vi "Agilent SNA Preset.vi"(7 "Agilent SNA & SWP":T1, 8 "error in (no error)":errorcluster, 11 "VISA Resource Names":T2) -> (0 "error out":errorcluster, 3 "dup VISA Resource Names":T2)   [LabVIEW 2011]
uses:
  TypeDefs/Agilent SNA VISA.ctl
  TypeDefs/Agilent SNA Instrument Info.ctl
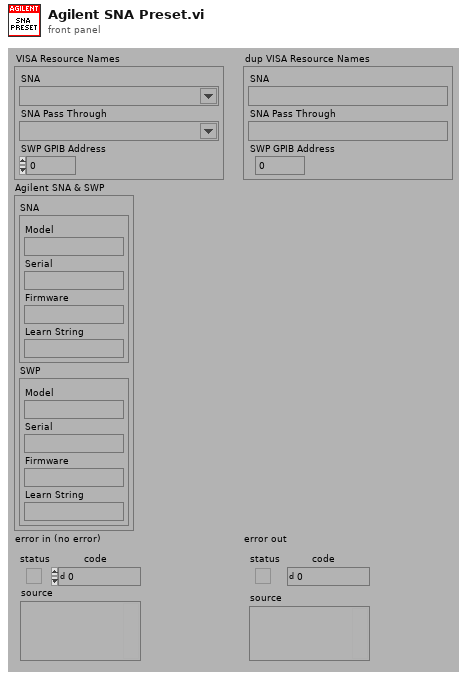
[diagram p1: front panel]
types:
  T1 = typedef "Agilent SNA Instrument Info.ctl" = cluster{"SNA":cluster{"Model":string, "Serial":string, "Firmware":string, "Learn String":string}, "SWP":cluster{"Model":string, "Serial":string, "Firmware":string, "Learn String":string}}
  T2 = typedef "Agilent SNA VISA.ctl" = cluster{"SNA":refnum<visa-resource-name>, "SNA Pass Through":refnum<visa-resource-name>, "SWP GPIB Address":i32}
  T3 = typedef "Agilent SNA Model.ctl" = enum16{"Not Supported", "8757X"}
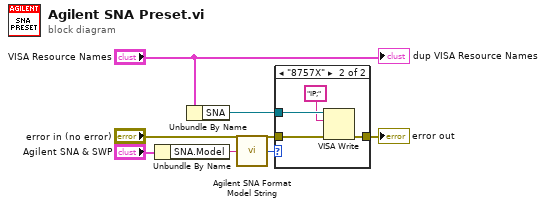
[diagram p0: block diagram]
diagram:
  n1 = Unbundle By Name("Agilent SNA & SWP") -> ("SNA.Model"=w3:string)
  n2 = Unbundle By Name("VISA Resource Names") -> ("SNA"=w2:refnum<visa-resource-name>)
  n3 = call "Agilent SNA Format Model String.vi"("Model String"=w3) -> ("Model"=w5:T3)
  n4 = case shown="\"8757X\"" w5 {
    tunnel: "error in (no error)" -> [w8 w12]
    tunnel: w2 -> [_ w11]
    tunnel: [w8 w10] -> w6
    frame "Not Supported" {
    }
    frame "8757X" {
      n5 = VISA Write(VISA resource name=w11, write buffer="IP;", error in (no error)=w12) -> (error out=w10:errorcluster)  [unwired: 2 out]
    }
  }
  "error out" <- w6
  "dup VISA Resource Names" <- "VISA Resource Names"
